vi "SPI RX bit.vi"(7 "CPOL":bool=TRUE, 11 "I/O Cluster In":T1) -> (1 "Signal":bool, 3 "I/O Cluster Out":T1)   [LabVIEW 2016, in "jmslib.lvlib"]
uses:
  jmslib.lvlib
  <vilib>/rvi/eio/common/nirviEmuTemplateMethod_errors.vi
  <vilib>/eio/EIONode/EIONode.xnode
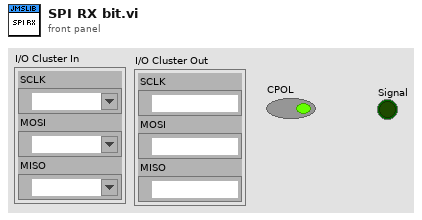
[diagram p1: front panel]
types:
  T1 = cluster{"SCLK":refnum<k21>, "MOSI":refnum<k21>, "MISO":refnum<k21>}
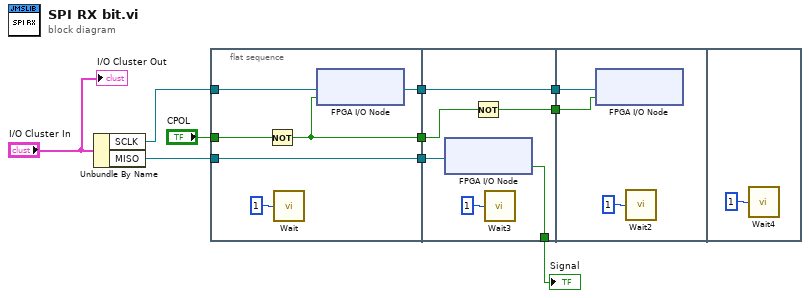
[diagram p0: block diagram]
diagram:
  n1 = Unbundle By Name("I/O Cluster In") -> ("SCLK"=w3:refnum<k21>, "MISO"=w2:refnum<k21>)
  n2 = flat-sequence {
    tunnel: "CPOL" -> [w12]
    tunnel: w3 -> [w15]
    tunnel: w2 -> [w13]
    tunnel: [w14] -> w8
    tunnel: [w13] -> w7
    tunnel: [w11] -> w5
    tunnel: [w21] -> w9
    tunnel: w8 -> [w21]
    tunnel: w7 -> [w20]
    tunnel: [w19] -> w6
    tunnel: w5 -> [w18]
    tunnel: [w17] -> w4
    tunnel: w9 -> [w23]
    tunnel: w4 -> [w24]
    frame #0 {
      n3 = Not(x=w12) -> (.not. x?=w11:bool)
      n4 = call "Wait"("Count(uSec)"=u16 1) -> ()  [unwired: 1 out]
      n5 = xnode "FPGA I/O Node"("I/O Item"=w11, "FPGA I/O In"=w15) -> ("FPGA I/O Out"=w14:refnum<k21>)
    }
    frame #1 {
      n6 = xnode "FPGA I/O Node"("FPGA I/O In"=w20) -> ("I/O Item"=w19:bool)  [unwired: 1 out]
      n7 = Not(x=w18) -> (.not. x?=w17:bool)
      n8 = call "Wait3"("Count(uSec)"=u16 1) -> ()  [unwired: 1 out]
    }
    frame #2 {
      n9 = xnode "FPGA I/O Node"("I/O Item"=w24, "FPGA I/O In"=w23) -> ()  [unwired: 1 out]
      n10 = call "Wait2"("Count(uSec)"=u16 1) -> ()  [unwired: 1 out]
    }
    frame #3 {
      n11 = call "Wait4"("Count(uSec)"=u16 1) -> ()  [unwired: 1 out]
    }
  }
  "Signal" <- w6
  "I/O Cluster Out" <- "I/O Cluster In"
